vi "FindVirtualFolders.vi"(8 "error in (no error)":errorcluster, 11 "Name":string="Folder") -> (0 "error out":errorcluster, 2 "Found":bool, 3 "Folder":refnum<vi>)   [LabVIEW 2013, in "ProjectHandler.lvlib"]
uses:
  ProjectHandler.lvlib
  RefNums.vi
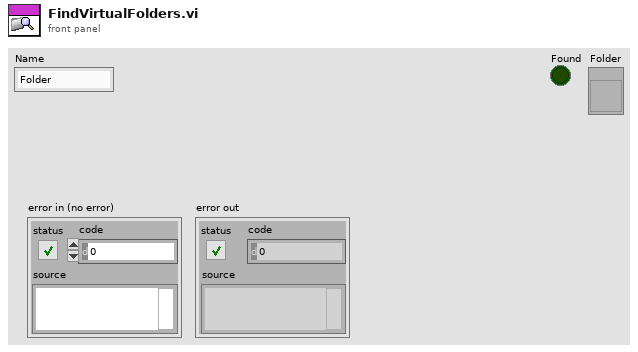
[diagram p1: front panel]
types:
  T1 = cluster{"App":refnum<vi>, "Project":refnum<vi>, "My Computer":refnum<vi>}
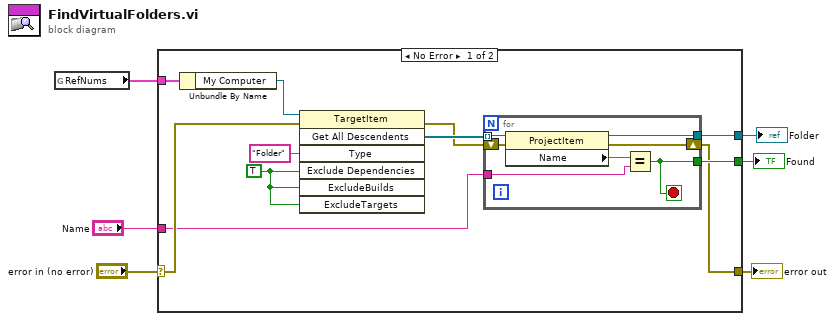
[diagram p0: block diagram]
diagram:
  n1 = global read "RefNums.vi" "RefNums"() -> (w4:T1)
  n2 = case shown="No Error" "error in (no error)" {
    selector: "error in (no error)" -> [w11 w25]
    tunnel: [w8 w25] -> w5
    tunnel: w4 -> [w17 _]
    tunnel: "Name" -> [w10 _]
    tunnel: [w9 _] -> w2
    tunnel: [w7 _] -> w1
    frame No Error {
      w15 = TRUE ("ExcludeDependencies")
      n3 = Unbundle By Name(w17) -> ("My Computer"=w12:refnum<vi>)
      n4 = invoke class="TargetItem" method="Get All Descendents"(reference=w12, error in=w11, "Type"="Folder", "Exclude Dependencies"=w15, "ExcludeBuilds"=w15, "ExcludeTargets"=w15) -> (error out=w13:errorcluster, "All Descendents"=w14:refnum<vi>[])  [unwired: 1 in, 5 out]
      n5 = for {
        tunnel: w14 -> [w24] mode=indexing
        tunnel: [w22] -> w9
        shift-right: [w21] -> w8
        shift-left: w13 -> [w20]
        tunnel: [w19] -> w7
        tunnel: w10 -> [w18]
        stop <- w22 stop-if-true
        n6 = property class="ProjectItem"(reference=w24, error in=w20) -> (reference out=w19:refnum<vi>, error out=w21:errorcluster, "Name"=w23:string)
        n7 = Equal?(x=w23, y=w18) -> (x = y?=w22:bool)
      }
    }
    frame Error {
    }
  }
  "error out" <- w5
  "Found" <- w2
  "Folder" <- w1
